vi "Initialize File Parsing Interface.vi"(8 "error in (no error)":errorcluster, 11 "niRFSTS Sequence Flow in":refnum<class "niRFSTS Sequence Flow.lvclass">) -> (0 "error out":errorcluster, 3 "niRFSTS Sequence Flow out":refnum<class "niRFSTS Sequence Flow.lvclass">)   [LabVIEW 2018, in "niRFSTS Sequence Flow.lvclass"]
uses:
  niRFSTS Sequence Flow.lvclass
  Plugins/File Parsing Interface.lvlibp/File Parsing Interface.lvclass
  niRFSTS Sequence Flow.lvclass/niRFSTS Sequence Flow.ctl
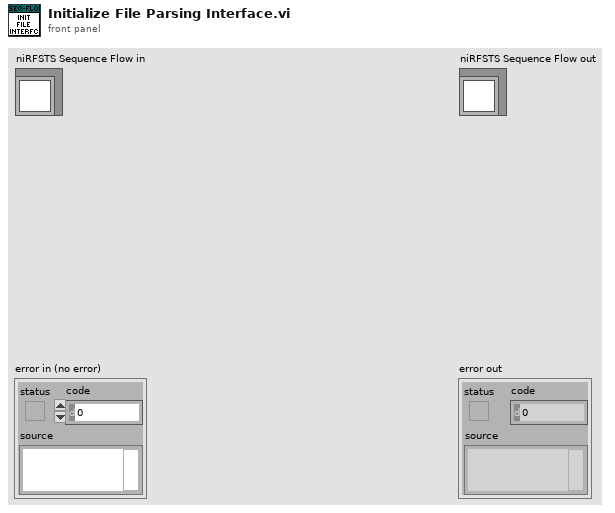
[diagram p1: front panel]
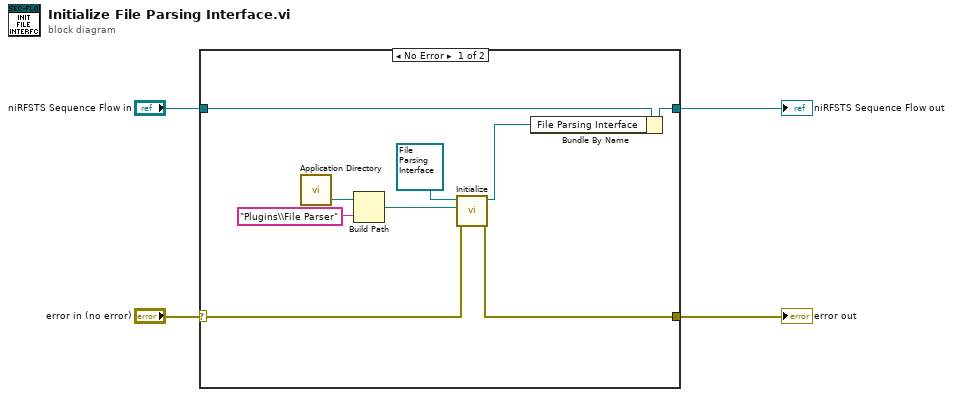
[diagram p0: block diagram]
diagram:
  n1 = case shown="No Error" "error in (no error)" {
    selector: "error in (no error)" -> [w8 w15]
    tunnel: [w7 w15] -> w3
    tunnel: [w6 w14] -> w1
    tunnel: "niRFSTS Sequence Flow in" -> [w13 w14]
    frame No Error {
      n2 = call <vilib>:"Application Directory.vi"() -> ("Application Directory"=w10:path)
      n3 = Build Path(base path=w10, name or relative path="Plugins\\File Parser") -> (appended path=w9:path)
      n4 = call-dynamic "Initialize.vi"("Error In"=w8, "Folder Path"=w9, "Plugin Framework In"=refnum<class "File Parsing Interface.lvclass"> refnum) -> ("Error Out"=w7:errorcluster, "File Parsing Interface out"=w5:refnum<class "File Parsing Interface.lvclass">)  [unwired: 7 in]
      n5 = Bundle By Name(cluster=w13, "File Parsing Interface"=w5) -> (w6:refnum<class "niRFSTS Sequence Flow.lvclass">)
    }
    frame Error {
    }
  }
  "error out" <- w3
  "niRFSTS Sequence Flow out" <- w1
